vi "USB_kernal_server.vi"(0 "Board type":T2=enum."NB-MIO-16H", 1 "Sync Mode?":bool, 2 "Client Time":dbl, 5 "No of samples+extra":i32=128 min=0 step=1, 7 "Trigger mode":T1, 9 "output polarity":u16(ring)=1 items=["do not change", "positive", "negative"], 11 "Ch & spans":T3[](array[typedef]) {"low limit (-10V)" format="%.3f"; "high limit (10V)" format="%.3f"}, 12 "Actual Sampling rate (Hz)":dbl=1000.0 format="%.2f", 13 "Local Client?":bool, 14 "Current Block No":i32) -> (4 "I16 data":i16[][](array[numeric]), 6 "Block Timings":T4={"Started"=0.0, "Ended"=0.0, "Analogue Frequency Hz"=1000.0} {"Analogue Frequency Hz" format="%.2f"}, 10 "group channel settings":T5(array[cluster]) {"scale offset" format="%.2f"; "scale multiplier" format="%.2f"; "gain" format="%.2f"; "range" format="%.2f"; "lower input limits" format="%.2f"; "upper input limits" format="%.2f"}, 15 "error out":errorcluster)   [LabVIEW 2010]
uses:
  Controls/Block_start_and_end.ctl
  Controls/Ch_and_Spans.ctl
  Controls/Board_Types.ctl
  Controls/Trigger_Mode.ctl
  PWA/PWAtasksGLOBAL.vi
  <vilib>/_DAQmxBase/Internals/DAQmxBase Timing (Sample Clock).vi
  <vilib>/_DAQmxBase/Internals/DAQmxBase Create Channel (AI-Voltage-Basic).vi
  Globals/Meas_global.vi
  Globals/LDA_meas_global_1.vi
  <vilib>/_DAQmxBase/Internals/DAQmxBase Read (Analog 2D DBL NChan NSamp).vi
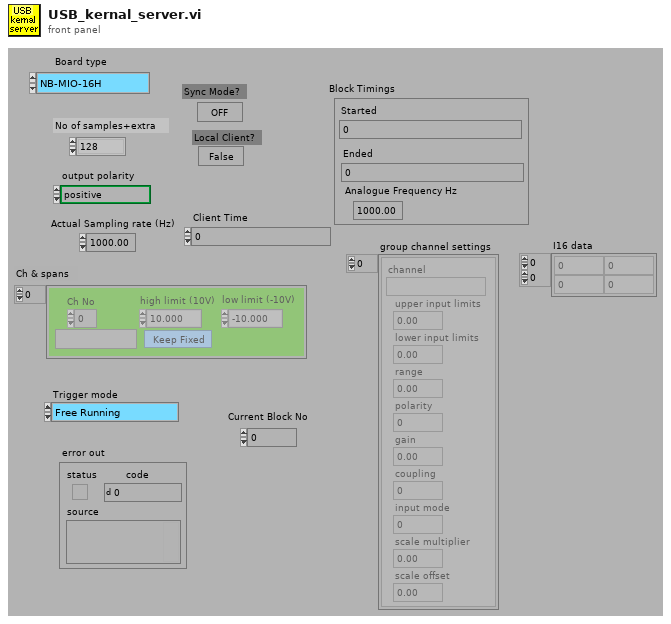
[diagram p1: front panel]
types:
  T1 = typedef "Trigger_Mode.ctl" = enum16{"Free Running", "Start on Trigger", "Trigger Every Block", "Trigger Every Sample"}
  T2 = typedef "Board_Types.ctl" = enum16{"Simulate", "NB-MIO-16H", "PCI-MIO-16E", "6000E Series", "USB-92xx", "ADC488", "Lab-NB", "NB-DIO-24", "NI-DAQmx", "Local ADAM", "Server Channels"}
  T3 = typedef "Ch_and_Spans.ctl" = cluster{"high limit (10V)":sgl, "low limit (-10V)":sgl, "Ch No":i16, "Var name":string, "Use Latest Calib":bool}
  T4 = typedef "Block_start_and_end.ctl" = cluster{"Started":dbl, "Ended":dbl, "Analogue Frequency Hz":dbl}
  T5 = cluster{"channel":string, "upper input limits":sgl, "lower input limits":sgl, "range":sgl, "polarity":u16, "gain":sgl, "coupling":u16, "input mode":u16, "scale multiplier":dbl, "scale offset":dbl}[]
  T6 = typedef "BSA_info_Cluster.ctl" = cluster{"GPIB Address":string, "No of Check Bytes":i32, "Extra Info":string, "COLOUR":u32, "Wavelength (nm)":dbl}
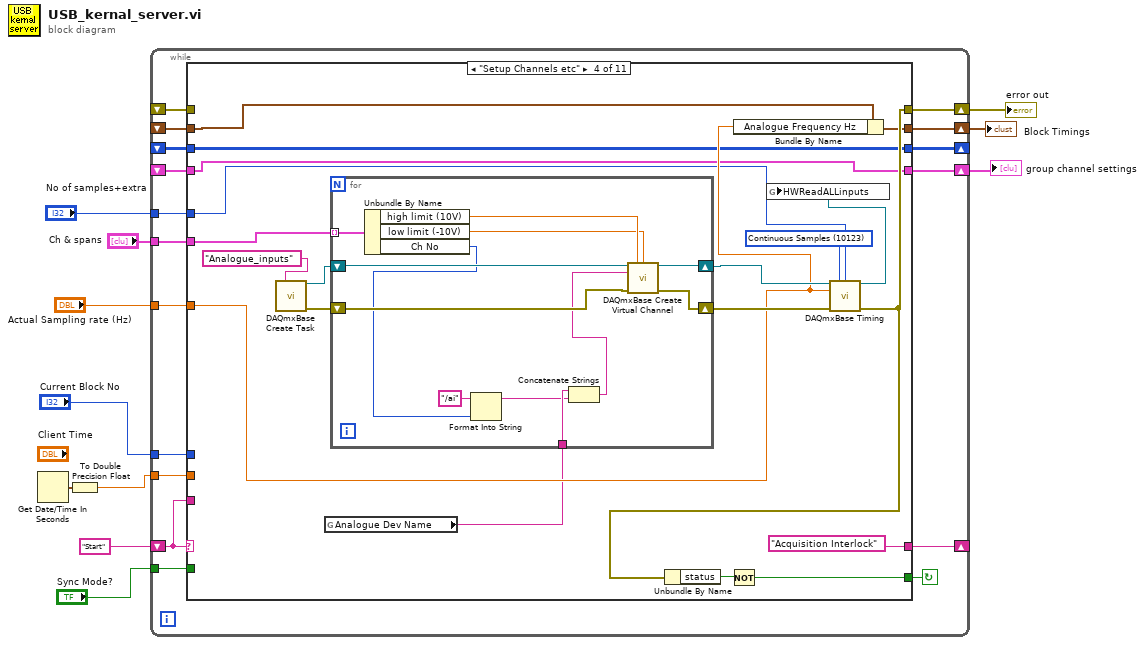
[diagram p0: block diagram]
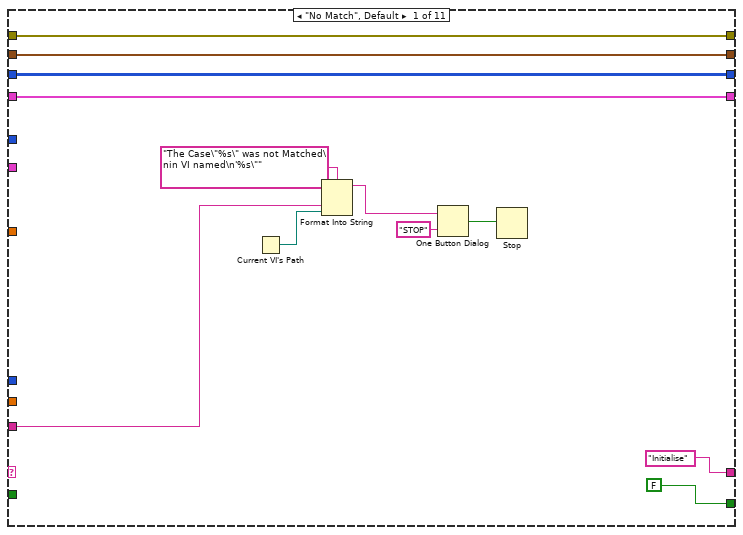
[diagram p2: hidden frame]
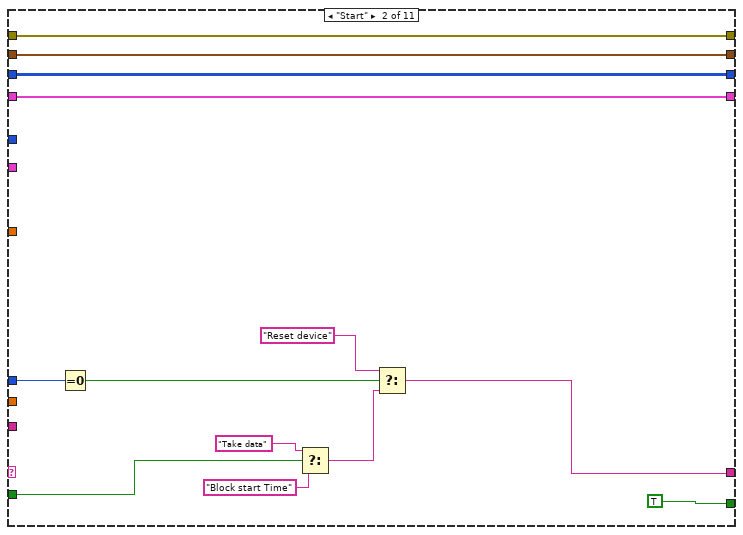
[diagram p3: hidden frame]
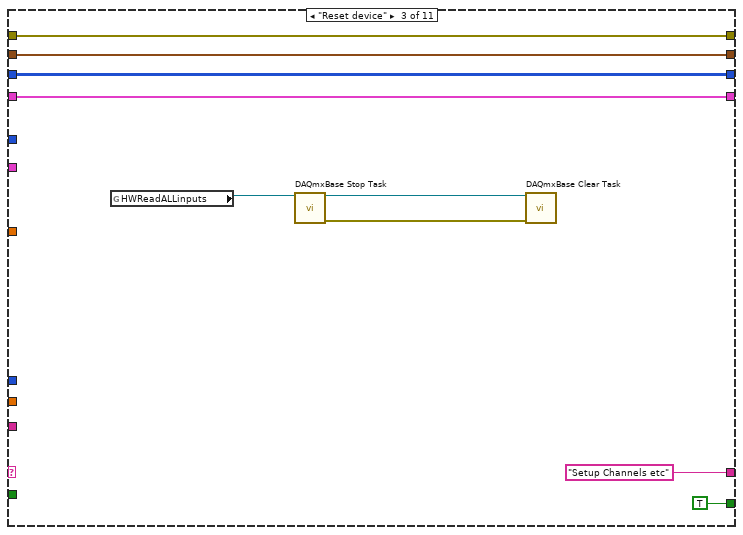
[diagram p4: hidden frame]
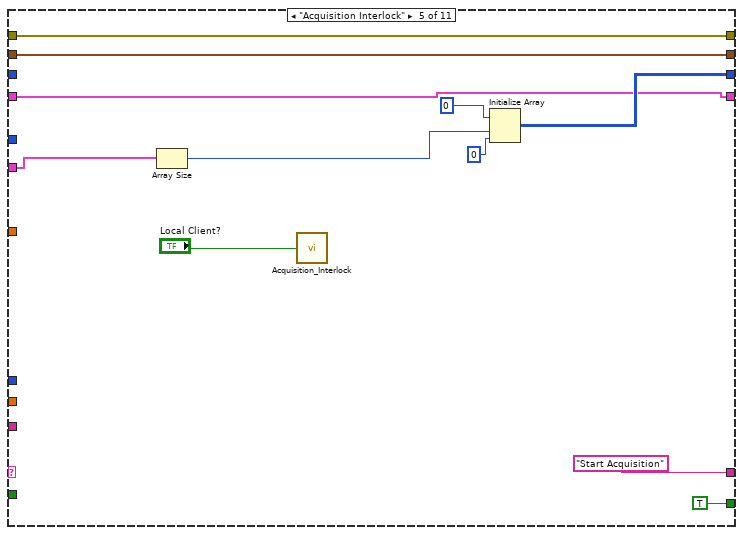
[diagram p5: hidden frame]
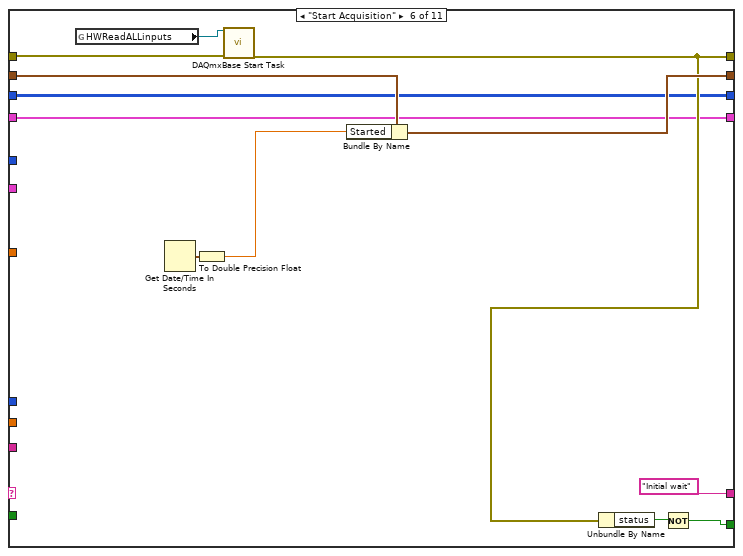
[diagram p6: hidden frame]
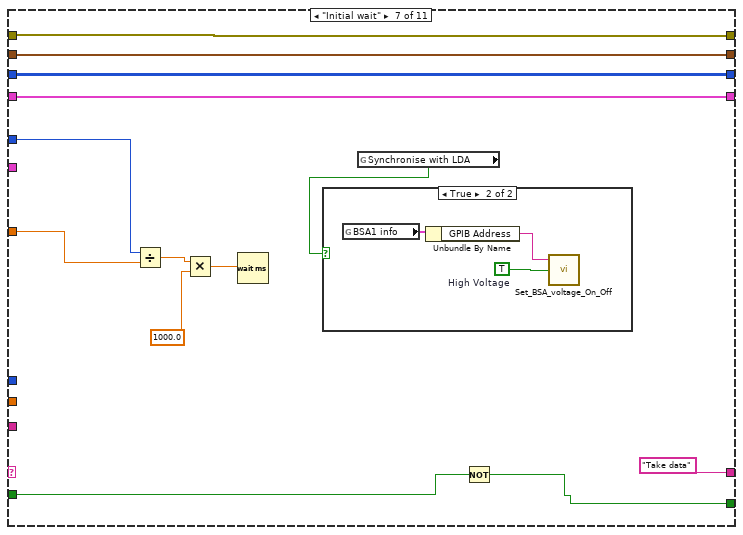
[diagram p7: hidden frame]
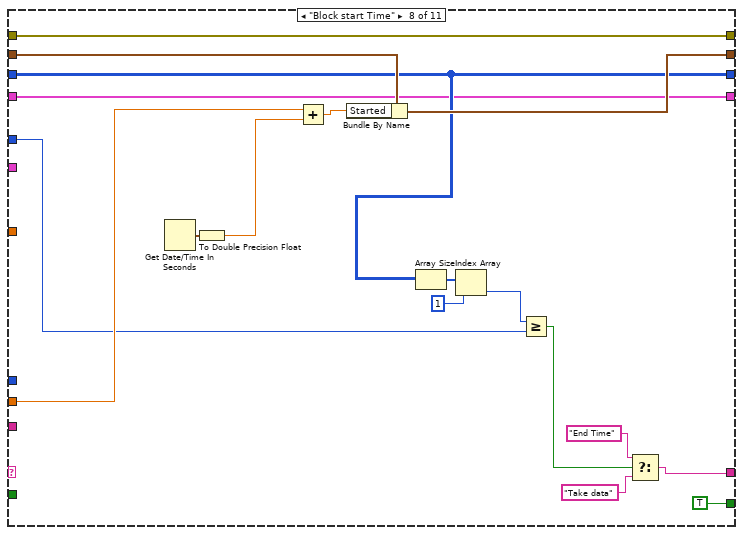
[diagram p9: hidden frame]
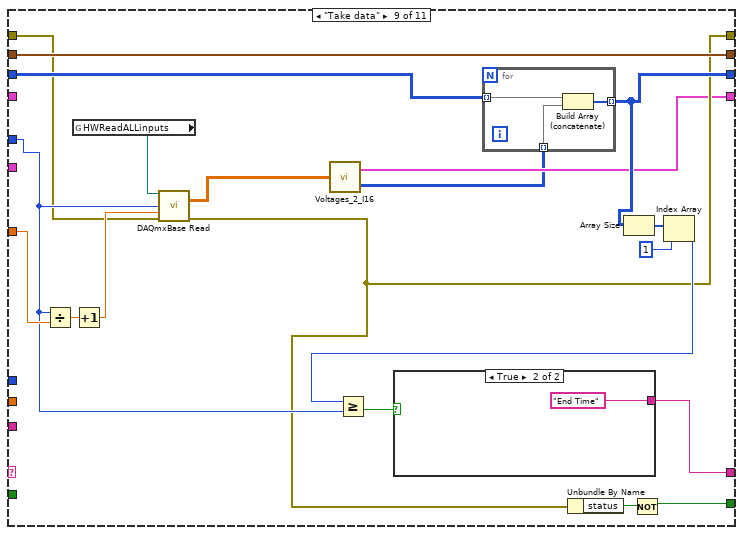
[diagram p10: hidden frame]
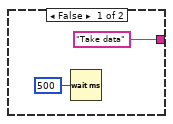
[diagram p11: hidden frame]
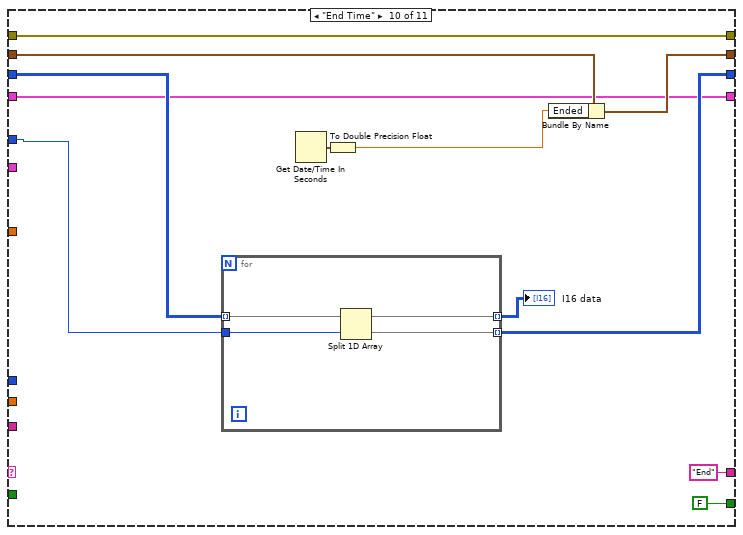
[diagram p12: hidden frame]
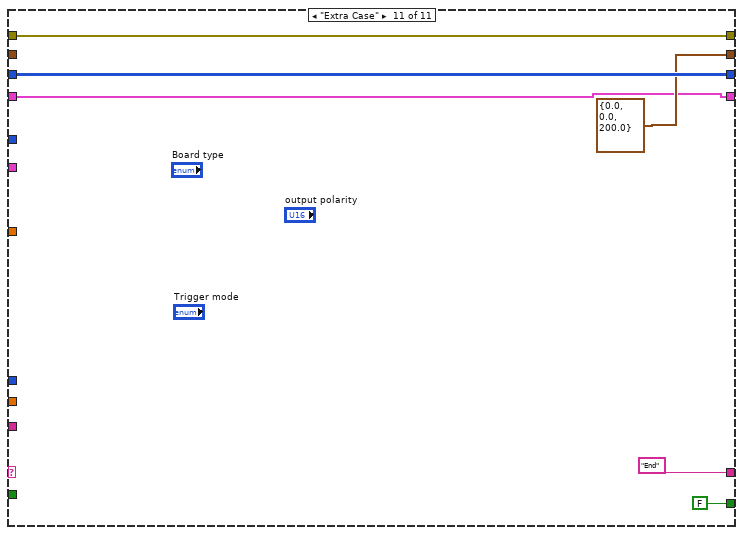
[diagram p13: hidden frame]
diagram:
  n1 = Get Date/Time In Seconds() -> (seconds since 1Jan1904=w10:timestamp)
  n2 = To Double Precision Float(number=w10) -> (double precision float=w1:dbl)
  n3 = while {
    shift-left: "Start" -> [w26]
    shift-right: [w27] -> _
    shift-right: [w25] -> w9
    shift-left: _ -> [w24]
    shift-right: [w23] -> w8
    shift-left: _ -> [w22]
    tunnel: w1 -> [w21]
    tunnel: "Actual Sampling rate (Hz)" -> [w20]
    tunnel: "No of samples+extra" -> [w19]
    shift-right: [w16] -> _
    shift-left: _ -> [w17]
    tunnel: "Current Block No" -> [w18]
    tunnel: "Ch & spans" -> [w15]
    shift-right: [w14] -> w3
    shift-left: _ -> [w13]
    tunnel: "Sync Mode?" -> [w12]
    stop <- w28 continue-if-true
    n4 = case shown="\"Setup Channels etc\"" w26 {
      tunnel: [FALSE TRUE TRUE w73 TRUE w110 w118 TRUE w159 FALSE FALSE] -> w28
      tunnel: ["Initialise" w46 "Setup Channels etc" "Acquisition Interlock" "Start Acquisition" "Initial wait" "Take data" w135 w162 "End" ("f") "End"] -> w27
      tunnel: w26 -> [w35 _ _ _ _ _ _ _ _ _ _]
      tunnel: [w32 w52 w58 w75 w102 w109 w127 w144 w154 w188 w197] -> w25
      tunnel: w24 -> [w32 w52 w58 _ w102 w112 w127 w144 w155 w188 w197]
      tunnel: [w31 w51 w61 w71 w100 w113 w126 w148 w170 w184 T4 {"Started"=0.0, "Ended"=0.0, "Analogue Frequency Hz"=200.0} ("Block Timings")] -> w23
      tunnel: w22 -> [w31 w51 w61 w72 w100 w114 w126 w149 w170 w185 _]
      tunnel: w21 -> [_ _ _ _ _ _ _ w146 _ _ _]
      tunnel: w20 -> [_ _ _ w70 _ _ w124 _ w169 _ _]
      tunnel: w19 -> [_ _ _ w69 _ _ w125 w138 w157 w183 _]
      tunnel: w18 -> [_ w49 _ _ _ _ _ _ _ _ _]
      tunnel: w17 -> [w30 w50 w57 w67 _ w108 w128 w140 w167 w182 w195]
      tunnel: [w30 w50 w57 w67 w95 w108 w128 w140 w166 w180 w195] -> w16
      tunnel: w15 -> [_ _ _ w68 w98 _ _ _ _ _ _]
      tunnel: [w29 w45 w55 w66 w94 w107 w120 w133 w153 w178 w193] -> w14
      tunnel: w13 -> [w29 w45 w55 w66 w94 w107 w120 w133 _ w178 w193]
      tunnel: w12 -> [_ w44 _ _ _ _ w117 _ _ _ _]
      frame "No Match", Default {
        n5 = Current VI's Path() -> (path=w34:path)
        n6 = Format Into String(format string="The Case\"%s\" was not Matched\nin VI named\n'%s\"" ("Format String"), w35, w34) -> (resulting string=w38:string)  [unwired: 2 in, 1 out]
        n7 = One Button Dialog(message=w38, button name ("OK")="STOP") -> (true=w36:bool)
        n8 = Stop(stop? (T)=w36) -> ()
      }
      frame "Start" {
        n9 = Equal To 0?(x=w49) -> (x = 0?=w47:bool)
        n10 = Select(t="Take data", s=w44, f="Block start Time") -> (s? t:f=w43:string)
        n11 = Select(t="Reset device", s=w47, f=w43) -> (s? t:f=w46:string)
      }
      frame "Reset device" {
        n12 = global read "PWAtasksGLOBAL.vi" "HWReadALLinputs"() -> (w54:refnum<k21>)
        n13 = call <vilib>:"DAQmxBase Stop Task.vi"("task/channels in"=w54) -> ("task out"=w60:refnum<k21>, "error out"=w59:errorcluster)  [unwired: 13 in]
        n14 = call <vilib>:"DAQmxBase Clear Task.vi"("task in"=w60, "error in"=w59) -> ()  [unwired: 13 in, 1 out]
      }
      frame "Setup Channels etc" {
        w78 = 10123 items=["Finite Samples"=10178, "Continuous Samples"=10123, "Hardware Timed Single Point"=12522] ("sample mode")
        n15 = call <vilib>:"DAQmxBase Create Task.vi"("new task name"="Analogue_inputs") -> ("task out"=w76:refnum<k21>, "error out"=w79:errorcluster)  [unwired: 13 in]
        n16 = global read "PWAtasksGLOBAL.vi" "Analogue Dev Name"() -> (w63:string)
        n17 = for {
          tunnel: w68 -> [w93] mode=indexing
          shift-right: [w89] -> w77
          shift-left: w76 -> [w90]
          shift-right: [w87] -> w80
          shift-left: w79 -> [w88]
          tunnel: w63 -> [w86]
          n18 = Unbundle By Name(w93) -> ("high limit (10V)"=w92:sgl, "low limit (-10V)"=w91:sgl, "Ch No"=w84:i16)
          n19 = Format Into String(initial string="/ai", w84) -> (resulting string=w82:string)  [unwired: 2 in, 1 out]
          n20 = Concatenate Strings(w86, w82) -> (w85:string)
          n21 = call-poly <vilib>:"DAQmxBase Create Virtual Channel.vi"("task in"=w90, "maximum value"=w92, "minimum value"=w91, "physical channels"=w85, "error in"=w88) -> ("task out"=w89:refnum<k21>, "error out"=w87:errorcluster)  [unwired: 9 in]
        }
        n22 = Bundle By Name(cluster=w72, "Analogue Frequency Hz"=w70) -> (w71:T4)
        n23 = call-poly <vilib>:"DAQmxBase Timing.vi"("task/channels in"=w77, "sample mode"=w78, "samples per channel"=w69, "rate"=w70, "error in"=w80) -> ("task out"=w64:refnum<k21>, "error out"=w75:errorcluster)  [unwired: 9 in]
        n24 = Unbundle By Name(w75) -> ("status"=w74:bool)
        n25 = Not(x=w74) -> (.not. x?=w73:bool)
        n26 = global write "PWAtasksGLOBAL.vi" "HWReadALLinputs"(w64) -> ()
      }
      frame "Acquisition Interlock" {
        n27 = Array Size(array=w98) -> (size(s)=w97:i32)
        n28 = call "Acquisition_Interlock.vi"("Local Control"="Local Client?") -> ()
        n29 = Initialize Array(i16 0, w97, 0 ("dimension size")) -> (w95:i16[][])
      }
      frame "Start Acquisition" {
        n30 = global read "PWAtasksGLOBAL.vi" "HWReadALLinputs"() -> (w106:refnum<k21>)
        n31 = Get Date/Time In Seconds() -> (seconds since 1Jan1904=w115:timestamp)
        n32 = To Double Precision Float(number=w115) -> (double precision float=w105:dbl)
        n33 = call <vilib>:"DAQmxBase Start Task.vi"("task/channels in"=w106, "error in"=w112) -> ("error out"=w109:errorcluster)  [unwired: 12 in, 1 out]
        n34 = Bundle By Name(cluster=w114, "Started"=w105) -> (w113:T4)
        n35 = Unbundle By Name(w109) -> ("status"=w111:bool)
        n36 = Not(x=w111) -> (.not. x?=w110:bool)
      }
      frame "Initial wait" {
        n37 = Divide(x=w125, y=w124) -> (x/y=w123:dbl)
        n38 = Multiply(x=w123, y=1000.0) -> (x*y=w121:dbl)
        n39 = Wait (ms)(milliseconds to wait=w121) -> ()  [unwired: 1 out]
        n40 = global read "Meas_global.vi" "Synchronise with LDA"() -> (w119:bool)
        n41 = case shown="True" w119 {
          frame False {
          }
          frame True {
            w130 = TRUE  # High Voltage
            n42 = global read "LDA_meas_global_1.vi" "BSA1 info"() -> (w131:T6)
            n43 = Unbundle By Name(w131) -> ("GPIB Address"=w132:string)
            n44 = call "Set_BSA_voltage_On_Off.vi"("GPIB address"=w132, "High Voltage"=w130) -> ()  [unwired: 5 in, 1 out]
          }
        }
        n45 = Not(x=w117) -> (.not. x?=w118:bool)
      }
      frame "Block start Time" {
        n46 = Get Date/Time In Seconds() -> (seconds since 1Jan1904=w150:timestamp)
        n47 = To Double Precision Float(number=w150) -> (double precision float=w147:dbl)
        n48 = Add(x=w146, y=w147) -> (x+y=w145:dbl)
        n49 = Bundle By Name(cluster=w149, "Started"=w145) -> (w148:T4)
        n50 = Array Size(array=w140) -> (size(s)=w142:i32[])
        n51 = Index Array(array=w142, index=1) -> (element=w139:i32)
        n52 = Greater Or Equal?(x=w139, y=w138) -> (x >= y?=w137:bool)
        n53 = Select(t="End Time", s=w137, f="Take data") -> (s? t:f=w135:string)
      }
      frame "Take data" {
        n54 = Divide(x=w157, y=w169) -> (x/y=w168:dbl)
        n55 = global read "PWAtasksGLOBAL.vi" "HWReadALLinputs"() -> (w158:refnum<k21>)
        n56 = Increment(x=w168) -> (x+1=w156:dbl)
        n57 = call-poly <vilib>:"DAQmxBase Read.vi"("task/channels in"=w158, "number of samples per channel"=w157, "timeout"=w156, "error in"=w155) -> ("data"=w151:dbl[][], "error out"=w154:errorcluster)  [unwired: 9 in, 1 out]
        n58 = call "Voltages_2_I16.vi"("Voltages"=w151) -> ("Group Channel Settings"=w153:T5, "I16 data"=w152:i16[][])
        n59 = for {
          tunnel: w152 -> [w176] mode=indexing
          tunnel: w167 -> [w175] mode=indexing
          tunnel: [w174] -> w166 mode=indexing
          n60 = Build Array (concatenate)(w175, w176) -> (w174:i16[])
        }
        n61 = Unbundle By Name(w154) -> ("status"=w160:bool)
        n62 = Array Size(array=w166) -> (size(s)=w165:i32[])
        n63 = Not(x=w160) -> (.not. x?=w159:bool)
        n64 = Index Array(array=w165, index=1) -> (element=w163:i32)
        n65 = Greater Or Equal?(x=w163, y=w157) -> (x >= y?=w161:bool)
        n66 = case shown="True" w161 {
          tunnel: ["Take data" "End Time"] -> w162
          frame False {
            n67 = Wait (ms)(milliseconds to wait=u32 500) -> ()  [unwired: 1 out]
          }
          frame True {
          }
        }
      }
      frame "End Time" {
        n68 = for {
          tunnel: w182 -> [w192] mode=indexing
          tunnel: w183 -> [w191]
          tunnel: [w190] -> w179 mode=indexing
          tunnel: [w189] -> w180 mode=indexing
          n69 = Split 1D Array(array=w192, index=w191) -> (first subarray=w190:i16[], second subarray=w189:i16[])
        }
        "I16 data" <- w179
        n70 = Get Date/Time In Seconds() -> (seconds since 1Jan1904=w186:timestamp)
        n71 = To Double Precision Float(number=w186) -> (double precision float=w177:dbl)
        n72 = Bundle By Name(cluster=w185, "Ended"=w177) -> (w184:T4)
      }
      frame "Extra Case" {
      }
    }
  }
  "error out" <- w9
  "Block Timings" <- w8
  "group channel settings" <- w3
